vi "EFMC-4.vi"(0 "数组":u8[](array[numeric])) -> (2 "地向加速度":i32, 3 "俯仰角速率":i16, 4 "滚转角速率":i16, 6 "东向加速度":i32, 8 "航向角速率":i16, 10 "北向加速度":i32, 12 "法向过载":i16, 13 "轴向过载":i16, 14 "侧向过载":i16)   [LabVIEW 2012]
uses:
  index-i32.vi
  XX-I32.vi
  index-i16.vi
  XX-I16.vi
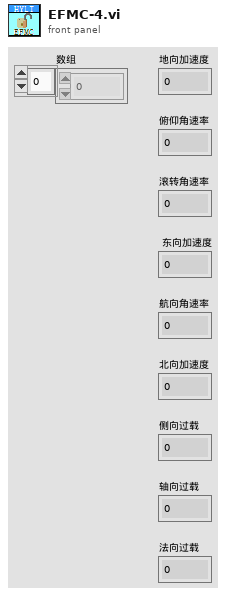
[diagram p1: front panel]
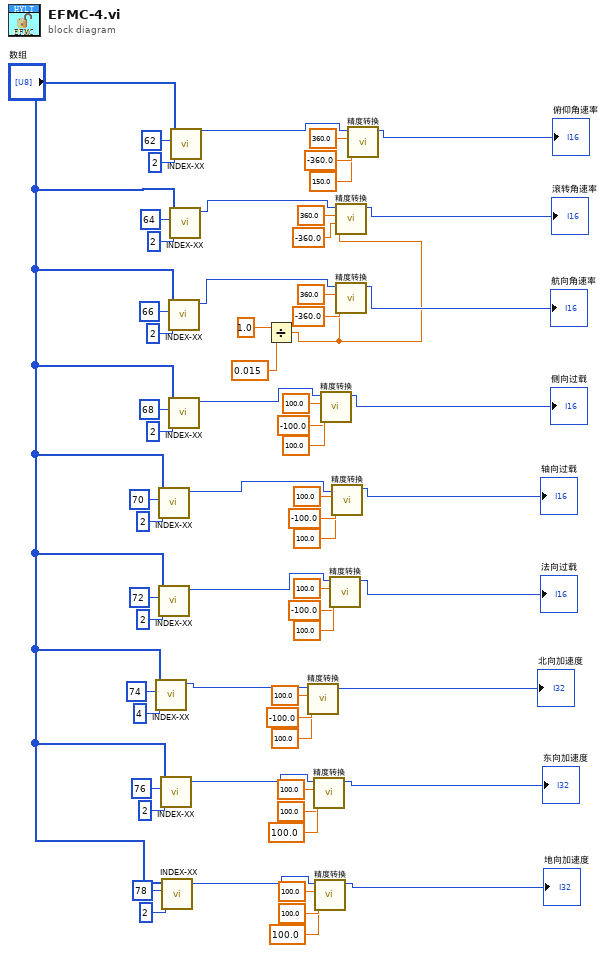
[diagram p0: block diagram]
diagram:
  n1 = call-poly "INDEX-XX.vi"("长度"=4, "索引"=74, "数组"="数组") -> ("数值输出"=w42:i32)  [unwired: 8 in]
  n2 = call-poly "INDEX-XX.vi"("长度"=2, "索引"=70, "数组"="数组") -> ("数值输出"=w11:i16)  [unwired: 8 in]
  n3 = call-poly "INDEX-XX.vi"("长度"=2, "索引"=72, "数组"="数组") -> ("数值输出"=w6:i16)  [unwired: 8 in]
  n4 = call-poly "INDEX-XX.vi"("长度"=2, "索引"=76, "数组"="数组") -> ("数值输出"=w33:i32)  [unwired: 8 in]
  n5 = call-poly "INDEX-XX.vi"("长度"=2, "索引"=78, "数组"="数组") -> ("数值输出"=w63:i32)  [unwired: 8 in]
  n6 = call-poly "INDEX-XX.vi"("长度"=2, "索引"=66, "数组"="数组") -> ("数值输出"=w21:i16)  [unwired: 8 in]
  n7 = call-poly "INDEX-XX.vi"("长度"=2, "索引"=68, "数组"="数组") -> ("数值输出"=w16:i16)  [unwired: 8 in]
  n8 = call-poly "INDEX-XX.vi"("长度"=2, "索引"=64, "数组"="数组") -> ("数值输出"=w25:i16)  [unwired: 8 in]
  n9 = call-poly "INDEX-XX.vi"("长度"=2, "索引"=62, "数组"="数组") -> ("数值输出"=w28:i32)  [unwired: 8 in]
  n10 = Divide(x=1.0, y=0.015 ("单位")) -> (x/y=w1:dbl)
  n11 = call-poly "精度转换.vi"("单位"=100.0, "下限"=-100.0, "上限"=100.0, "数值输入"=w42) -> ("输出"=→"北向加速度":i32)  [unwired: 7 in]
  n12 = call-poly "精度转换.vi"("单位"=100.0, "下限"=100.0, "上限"=100.0, "数值输入"=w33) -> ("输出"=→"东向加速度":i32)  [unwired: 7 in]
  n13 = call-poly "精度转换.vi"("单位"=100.0, "下限"=100.0, "上限"=100.0, "数值输入"=w63) -> ("输出"=→"地向加速度":i32)  [unwired: 7 in]
  n14 = call-poly "精度转换.vi"("单位"=100.0, "下限"=-100.0, "上限"=100.0, "数值输入"=w16) -> ("输出"=→"侧向过载":i16)  [unwired: 7 in]
  n15 = call-poly "精度转换.vi"("单位"=100.0, "下限"=-100.0, "上限"=100.0, "数值输入"=w6) -> ("输出"=→"法向过载":i16)  [unwired: 7 in]
  n16 = call-poly "精度转换.vi"("单位"=100.0, "下限"=-100.0, "上限"=100.0, "数值输入"=w11) -> ("输出"=→"轴向过载":i16)  [unwired: 7 in]
  n17 = call-poly "精度转换.vi"("单位"=w1, "下限"=-360.0, "上限"=360.0, "数值输入"=w25) -> ("输出"=→"滚转角速率":i16)  [unwired: 7 in]
  n18 = call-poly "精度转换.vi"("单位"=w1, "下限"=-360.0, "上限"=360.0, "数值输入"=w21) -> ("输出"=→"航向角速率":i16)  [unwired: 7 in]
  n19 = call-poly "精度转换.vi"("单位"=150.0, "下限"=-360.0, "上限"=360.0, "数值输入"=w28) -> ("输出"=→"俯仰角速率":i16)  [unwired: 7 in]
